vi "ExecuteCommand.vi"(8 "error in (no error)":errorcluster, 9 "taskId":i32(ring) items=["TLibrary", "T01", "T02", "T03", "T04", "T05", "T06", "T07", "T08", "T09", "T10", "T11", "T12", "T13", "T14", "T15", "T16", "T17", "T18", "T19", "T20", "T21", "T22", "T23", "T24", "T25", "T26", "T27", "T28", "T29", "T30", "T31"], 10 "Command Code":string, 11 "controller in":refnum<k24>) -> (0 "error out":errorcluster, 2 "return value":string, 3 "controller out":refnum<k24>)   [LabVIEW 2011]
uses:
  C:/Users/Admin/Desktop/Gantry Code Transfer/source/Code Transfer/Aerotech.A3200.dll
  Aerotech.A3200.dll
  C:/Users/Admin/Desktop/Gantry Code Transfer/source/Code Transfer/Aerotech.A3200.LabVIEW.dll
  Aerotech.A3200.LabVIEW.dll
panel:
  in  "Null":refnum<k24>
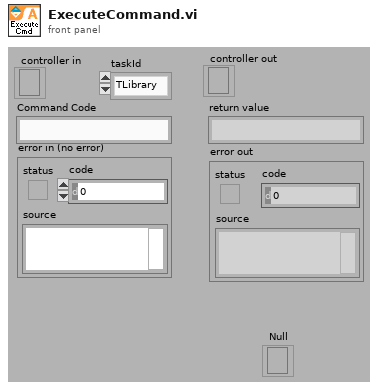
[diagram p1: front panel]
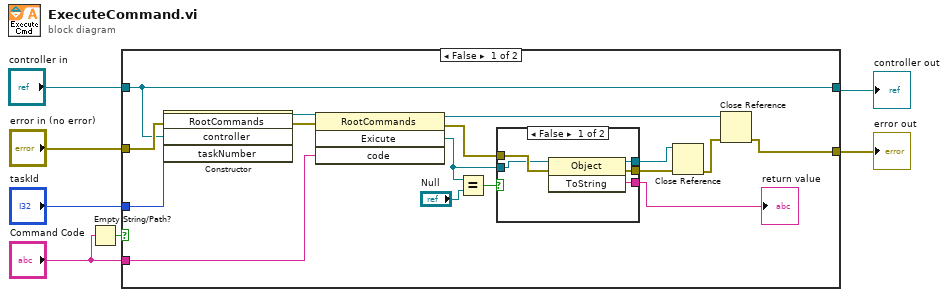
[diagram p0: block diagram]
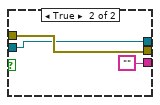
[diagram p2: hidden frame]
diagram:
  n1 = Empty String/Path?(string/path="Command Code") -> (empty?=w2:bool)
  n2 = case shown="False" w2 {
    tunnel: [w9 w32] -> w7
    tunnel: "error in (no error)" -> [w22 w32]
    tunnel: "controller in" -> [w18 w33]
    tunnel: "Command Code" -> [w20 _]
    tunnel: "taskId" -> [w19 _]
    tunnel: [w18 w33] -> w3
    frame False {
      n3 = constructor class="RootCommands"(error in=w22, "controller"=w18, "taskNumber"=w19) -> (reference out=w23:refnum<k24>, error out=w21:errorcluster)  [unwired: 2 in, 3 out]
      n4 = invoke class="RootCommands" method="Exicute"(reference=w23, error in=w21, "code"=w20) -> (reference out=w11:refnum<k24>, error out=w10:errorcluster, "Exicute"=w8:refnum<k24>)  [unwired: 1 in, 1 out]
      n5 = Equal?(x=w8, y="Null") -> (x = y?=w16:bool)
      n6 = case shown="False" w16 {
        tunnel: w10 -> [w28 w31]
        tunnel: [w27 w31] -> w13
        tunnel: w8 -> [w26 w29]
        tunnel: [w25 ""] -> w17
        tunnel: [w24 w29] -> w12
        frame False {
          n7 = invoke class="Object" method="ToString"(reference=w26, error in=w28) -> (reference out=w24:refnum<k24>, error out=w27:errorcluster, "ToString"=w25:string)  [unwired: 1 in]
        }
        frame True {
        }
      }
      "return value" <- w17
      n8 = Close Reference(reference=w12, error in (no error)=w13) -> (error out=w14:errorcluster)
      n9 = Close Reference(reference=w11, error in (no error)=w14) -> (error out=w9:errorcluster)
    }
    frame True {
    }
  }
  "error out" <- w7
  "controller out" <- w3
